vi "Initialization VI.vi"(8 "error in (no error)":errorcluster, 10 "Custom XML":string, 11 "Device Item Ref in":T1 format="%.0x") -> (0 "error out":errorcluster, 3 "Device Item Ref out":T1 format="%.0x")   [LabVIEW 2016, in "FPGA Resource Manager Client Example System Explorer.lvlib"]
uses:
  FPGA Resource Manager Client Example System Explorer.lvlib
  <vilib>/NI Veristand/Custom Device API/Custom Device Item Ref.ctl
  FPGA-Resource-Manager-APIs/Source/System Definition/API/Types/Channel Type.ctl
  FPGA-Resource-Manager-APIs/Source/Shared/FPGA RM Shared API.lvlib
  FPGA-Resource-Manager-APIs/Source/System Definition/FPGA RM System Definition API.lvlib
  <vilib>/NI VeriStand/Custom Device API/Custom Device API.lvlib
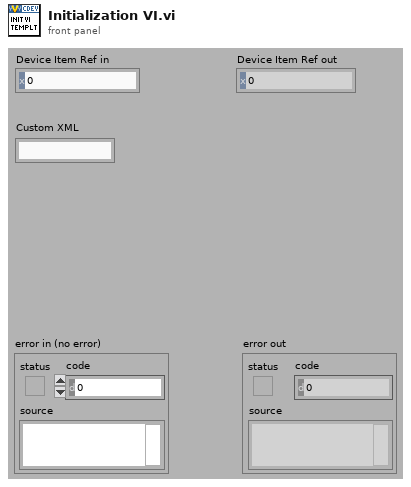
[diagram p1: front panel]
types:
  T1 = typedef "Custom Device API.lvlib/Custom Device Item Ref.ctl" = u64
  T2 = typedef "FPGA RM Shared API.lvlib/Channel Type.ctl" = enum16{"Write Channel", "Read Channel", "Write Waveform", "Read Waveform"}
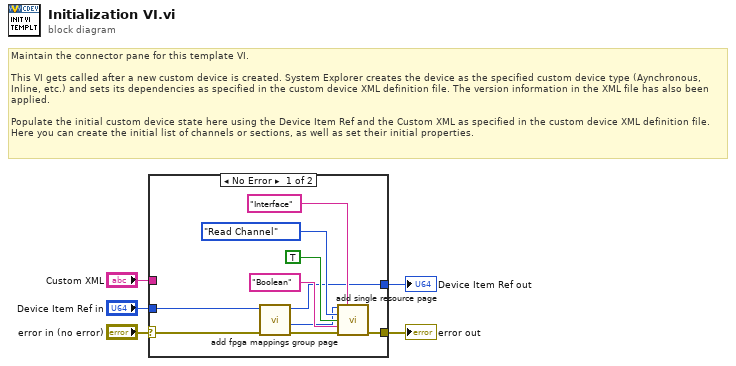
[diagram p0: block diagram]
diagram:
  # "Maintain the connector pane for this template VI.\n\nThis VI gets called after a new custom device is created. System Explorer creates the device as the specified custom device type (Aynchronous, Inline, etc.) and sets its dependencies as specified in the custom device XML definition file. The version information in the XML file has also been applied.\n\nPopulate the initial custom device state here using the Device Item Ref and the Custom XML as specified in the custom device XML definition file. Here you can create the initial list of channels or sections, as well as set their initial properties."
  n1 = case shown="No Error" "error in (no error)" {
    selector: "error in (no error)" -> [w8 w17]
    tunnel: [w14 w17] -> w5
    tunnel: [w6 w16] -> w3
    tunnel: "Device Item Ref in" -> [w15 w16]
    tunnel: "Custom XML" -> [_ _]
    frame No Error {
      n2 = call "add fpga mappings group page.vi"("error in (no error)"=w8, "Device Item Ref in"=w15) -> ("error out"=w7:errorcluster, "Section Ptr"=w9:T1, "Device Item Ref out"=w6:T1)  [unwired: 7 in]
      n3 = call "add single resource page.vi"("Section Ptr in"=w9, "cd resource name"="Interface", "channel type"=Channel_Type."Read Channel", "datatype"=TRUE, "name starts with..."="Boolean", "error in (no error)"=w7) -> ("error out"=w14:errorcluster)  [unwired: 8 in, 1 out]
    }
    frame Error {
    }
  }
  "error out" <- w5
  "Device Item Ref out" <- w3
